vi "Converte Floating Point - Hexadecimal IEEE 754.vi"(1 "Floating point (entrada)":sgl) -> (0 "Array 2*[U16]":u16[](array[numeric]))   [LabVIEW 2019]
doc: "Transforma um float single precision em 2 words [u16] de 16 bits segundo a norma IEEE 754"
panel:
  out "Float (confirmação)":sgl
  out "Mantissa":bool[](array[boolean])
  out "Array final":bool[](array[boolean])
  out "Sinal":bool[](array[boolean])
  out "Expoente":bool[](array[boolean])
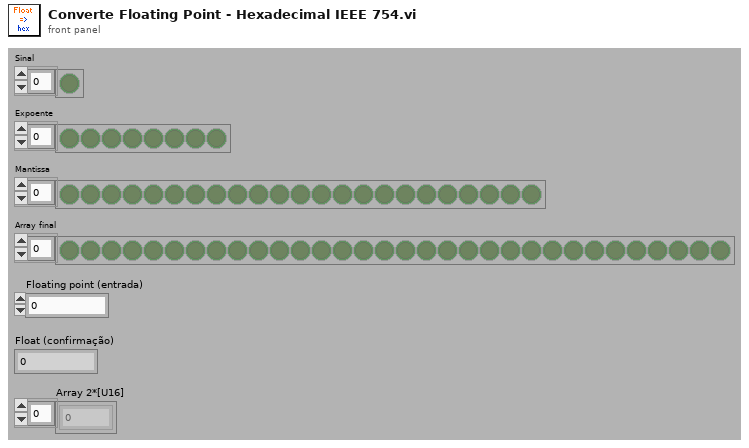
[diagram p1: front panel]
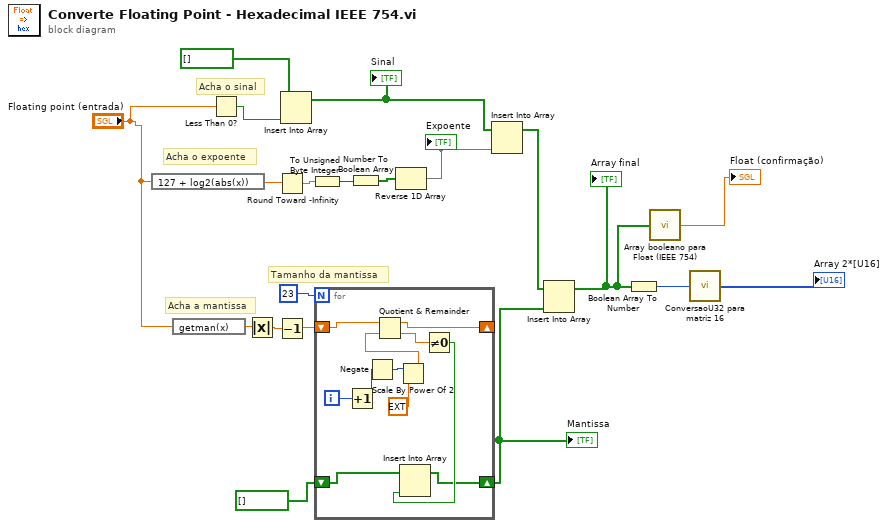
[diagram p0: block diagram]
diagram:
  # "Tamanho da mantissa"
  # "Acha o sinal"
  # "Acha o expoente"
  # "Acha a mantissa"
  n1 = expression code="127 + log2(abs(x))"("Floating point (entrada)") -> (w20:sgl)
  n2 = expression code="getman(x)"("Floating point (entrada)") -> (w5:sgl)
  n3 = Less Than 0?(x="Floating point (entrada)") -> (x < 0?=w19:bool)
  n4 = Absolute Value(x=w5) -> (abs(x)=w4:sgl)
  n5 = Round Toward -Infinity(1:w20) -> (0:w16:sgl)
  n6 = Decrement(x=w4) -> (x-1=w6:sgl)
  n7 = Insert Into Array(array=bool[] [], new element=w19) -> (w17:bool[])  [unwired: 1 in]
  "Sinal" <- w17
  n8 = To Unsigned Byte Integer(number=w16) -> (unsigned 8bit integer=w15:u8)
  n9 = for {
    N: 23 -> [_]
    shift-right: [w24] -> w11
    shift-left: bool[] [] ("Boolean array") -> [w26]
    shift-right: [w22] -> _
    shift-left: w6 -> [w23]
    i -> [w31]
    n10 = Increment(x=w31) -> (x+1=w21:i32)
    n11 = Negate(x=w21) -> (-x=w30:i32)
    n12 = Scale By Power Of 2(n=w30, x=ext 1.0) -> (x*2^n=w28:ext)
    n13 = Quotient & Remainder(x=w23, y=w28) -> (x-y*floor(x/y)=w22:ext, floor(x/y)=w27:ext)
    n14 = Not Equal To 0?(x=w27) -> (x != 0?=w25:bool)
    n15 = Insert Into Array(array=w26, new element=w25) -> (w24:bool[])  [unwired: 1 in]
  }
  "Mantissa" <- w11
  n16 = Number To Boolean Array(number=w15) -> (Boolean array=w8:bool[])
  n17 = Reverse 1D Array(array=w8) -> (reversed array=w7:bool[])
  "Expoente" <- w7
  n18 = Insert Into Array(array=w17, new element=w7) -> (w14:bool[])  [unwired: 1 in]
  n19 = Insert Into Array(array=w14, new element=w11) -> (w3:bool[])  [unwired: 1 in]
  "Array final" <- w3
  n20 = Boolean Array To Number(Boolean array=w3) -> (number=w2:u32)
  n21 = call "Array booleano para Float (IEEE 754).vi"("Array [32]"=w3) -> ("Float [SGL]"=→"Float (confirmação)":sgl)
  n22 = call "ConversaoU32 para matriz 16.vi"("Número [U32]"=w2) -> ("Array 2*[U16]"=→"Array 2*[U16]":u16[])
